vi "T2Mode_Acquisition_inertiaMotor.vi"() -> ()   [LabVIEW 2023]
uses:
  Types/MH_InputChannel.ctl
  Types/MH_UIThread_Cmds_T2.ctl
  cascorr/Multiharp/Types/MH_UIThread_Data_T2.ctl
  _lib/PQ/MultiHarp/MH_InitInfo.ctl
  Types/MH_SetInpChanData.ctl
  Types/MH_SetInpChanCmds.ctl
  _lib/PQ/MultiHarp/MH_RefSource.ctl
  _lib/PQ/MultiHarp/MH_MeasMode.ctl
  <vilib>/Utility/error.llb/DialogType.ctl
  <vilib>/Utility/error.llb/Error Cluster From Error Code.vi
  _lib/PQ/MultiHarp/MH_LibVersion_global.vi
  _lib/PQ/MultiHarp/mhlib_x86_x64_UIThread.llb/MH_DllPath_global.vi
  <vilib>/ErrorRing/Error Ring.xnode
panel:
  in  "Refresh(ms)":u32=500
  out "Waveform Chart":dbl[][](graph)
  in  "Monitor Range":i32=40
  in  "Path":path
  in  "FileName 2":string
  in  "Number of Acquisitions":i32=1 min=1 step=1
  out "x*y":dbl
  out "HistoGraph":T1(graph)={0.0, "Resolution"=0.08, "Histograms"=[]}
  in  "Run continuously":enum32{"Running Mode", "Item 1"}(radio) caption="Acquisition"
  in  "Start":bool
  in  "Scale":enum32{"Item 0", "Item 1"}(radio)
  out "CountRates":i32[](graph)
  in  "AllChannels":T2={"Enable"=TRUE, "Offset"=0, "Level"=20, "Edge"=0, "DeadTime"=1000, "UseDeadTime"=FALSE, "SetEnableAllChan"=TRUE, "SetEdgeAllChan"=TRUE, "SetLevelAllChan"=TRUE, "SetOffsetAllChan"=TRUE, "SetUseDTAllChan"=TRUE, "SetDeadTAllChan"=TRUE} {"DeadTime" min=800 max=160000 step=1; "Edge" items=["falling", "rising"]; "Offset" min=-100000 max=100000 step=10; "Level" min=-1200 max=1200 step=1}
  in  "HistoLength":i32(ring)=6 caption="Num Bins" items=["1024", "2048", "4096", "8192", "16384", "32768", "65536"]
  in  "OvlLevel":u32=4294967295 caption="Ovl.Level" min=1 step=1
  in  "StopOvl.":bool=TRUE
  in  "AcqTime":i32=1000 caption="Acqu.           ms" min=1 max=3600000 step=1
  in  "Binning":i32(ring) caption="Resol.            ps" items=["10", "20", "40", "80", "160", "320", "640", "1280", "2560", "5120", "10240", "20480", "40960", "81920", "163840", "327680", "655360", "1310720", "2621440", "5242880", "10485760", "20971520", "41943040"]
  in  "HistoOffset":i32 caption="Offset            ns" min=0 max=100000000 step=1
  in  "Acquire":bool
  in  "stop":bool
  in  "SyncDeadTime":i32=1000 caption="Dead T.   ps" min=800 max=160000 step=1
  in  "UseDeadTime":bool caption="Use DT."
  in  "SyncEdge":i32(ring) caption="Edge" items=["falling", "rising"]
  in  "SyncDivider":i32(ring) caption="Divider" items=["1", "2", "4", "8", "16"]
  in  "SyncOffset":i32 caption="Offset      ps" min=-100000 max=100000 step=10
  in  "SyncLevel":i32=-100 caption="Level      mV" min=-1200 max=1200 step=1
  in  "Channels":T3[](array[typedef])=[{"Name"="Inp.Chan 1", "Enable"=TRUE, "Edge"=0, "Level"=-100, "Offset"=0, "UseDeadTime"=FALSE, "DeadTime"=1000}, {"Name"="Inp.Chan 2", "Enable"=TRUE, "Edge"=0, "Level"=-100, "Offset"=0, "UseDeadTime"=FALSE, "DeadTime"=1000}, {"Name"="Inp.Chan 3", "Enable"=TRUE, "Edge"=0, "Level"=-100, "Offset"=0, "UseDeadTime"=FALSE, "DeadTime"=1000}, {"Name"="Inp.Chan 4", "Enable"=TRUE, "Edge"=0, "Level"=-100, "Offset"=0, "UseDeadTime"=FALSE, "DeadTime"=1000}, {"Name"="Inp.Chan 5", "Enable"=TRUE, "Edge"=0, "Level"=-100, "Offset"=0, "UseDeadTime"=FALSE, "DeadTime"=1000}, {"Name"="Inp.Chan 6", "Enable"=TRUE, "Edge"=0, "Level"=-100, "Offset"=0, "UseDeadTime"=FALSE, "DeadTime"=1000}, {"Name"="Inp.Chan 7", "Enable"=TRUE, "Edge"=0, "Level"=-100, "Offset"=0, "UseDeadTime"=FALSE, "DeadTime"=1000}, {"Name"="Inp.Chan 8", "Enable"=TRUE, "Edge"=0, "Level"=-100, "Offset"=0, "UseDeadTime"=FALSE, "DeadTime"=1000}, {"Name"="Inp.Chan 9", "Enable"=TRUE, "Edge"=0, "Level"=-100, "Offset"=0, "UseDeadTime"=FALSE, "DeadTime"=1000}, {"Name"="Inp.Chan 10", "Enable"=TRUE, "Edge"=0, "Level"=-100, "Offset"=0, "UseDeadTime"=FALSE, "DeadTime"=1000}, {"Name"="Inp.Chan 11", "Enable"=TRUE, "Edge"=0, "Level"=-100, "Offset"=0, "UseDeadTime"=FALSE, "DeadTime"=1000}, {"Name"="Inp.Chan 12", "Enable"=TRUE, "Edge"=0, "Level"=-100, "Offset"=0, "UseDeadTime"=FALSE, "DeadTime"=1000}, {"Name"="Inp.Chan 13", "Enable"=TRUE, "Edge"=0, "Level"=-100, "Offset"=0, "UseDeadTime"=FALSE, "DeadTime"=1000}, {"Name"="Inp.Chan 14", "Enable"=TRUE, "Edge"=0, "Level"=-100, "Offset"=0, "UseDeadTime"=FALSE, "DeadTime"=1000}, {"Name"="Inp.Chan 15", "Enable"=TRUE, "Edge"=0, "Level"=-100, "Offset"=0, "UseDeadTime"=FALSE, "DeadTime"=1000}, {"Name"="Inp.Chan 16", "Enable"=TRUE, "Edge"=0, "Level"=-100, "Offset"=0, "UseDeadTime"=FALSE, "DeadTime"=1000}] {"DeadTime" min=800 max=160000 step=1; "Edge" items=["falling", "rising"]; "Offset" min=-100000 max=100000 step=10; "Level" min=-1200 max=1200 step=1}
  out "SyncRate":string="Sync Rate: 4999950 cps\n"
  out "OverFlow":bool caption="Overflow:"
  out "Status":string="Readout Rate: 8.6 Hz\t\tTotal Counts:\t\tCh. 1: 0 cnts.\t\tCh. 2: 1962112 cnts.\t\tCh. 3: 0 cnts.\t\tCh. 4: 1962112 cnts.\t\tCh. 5: 0 cnts.\t\tCh. 6: 1962112 cnts.\t\tCh. 7: 0 cnts.\t\tCh. 8: 1962112 cnts.\t\tCh. 9: 1962113 cnts.\t\tCh.10: 0 cnts.\t\tCh.11: 1962113 cnts.\t\tCh.12: 0 cnts.\t\tCh.13: 1962113 cnts.\t\tCh.14: 0 cnts.\t\tCh.15: 1962113 cnts.\t\tCh.16: 1962113 cnts.\t\t"
  # "Single Counts"
  # "Coincidences vs time"
  # "Coincidences vs delay"
  # "Acquisition Options"
  # "Acquire Data"
  # "Piezo"
  # "Stage piezo"
  # "Scan"
  # "Jog"
  # "All Channels"
  # "Sync"
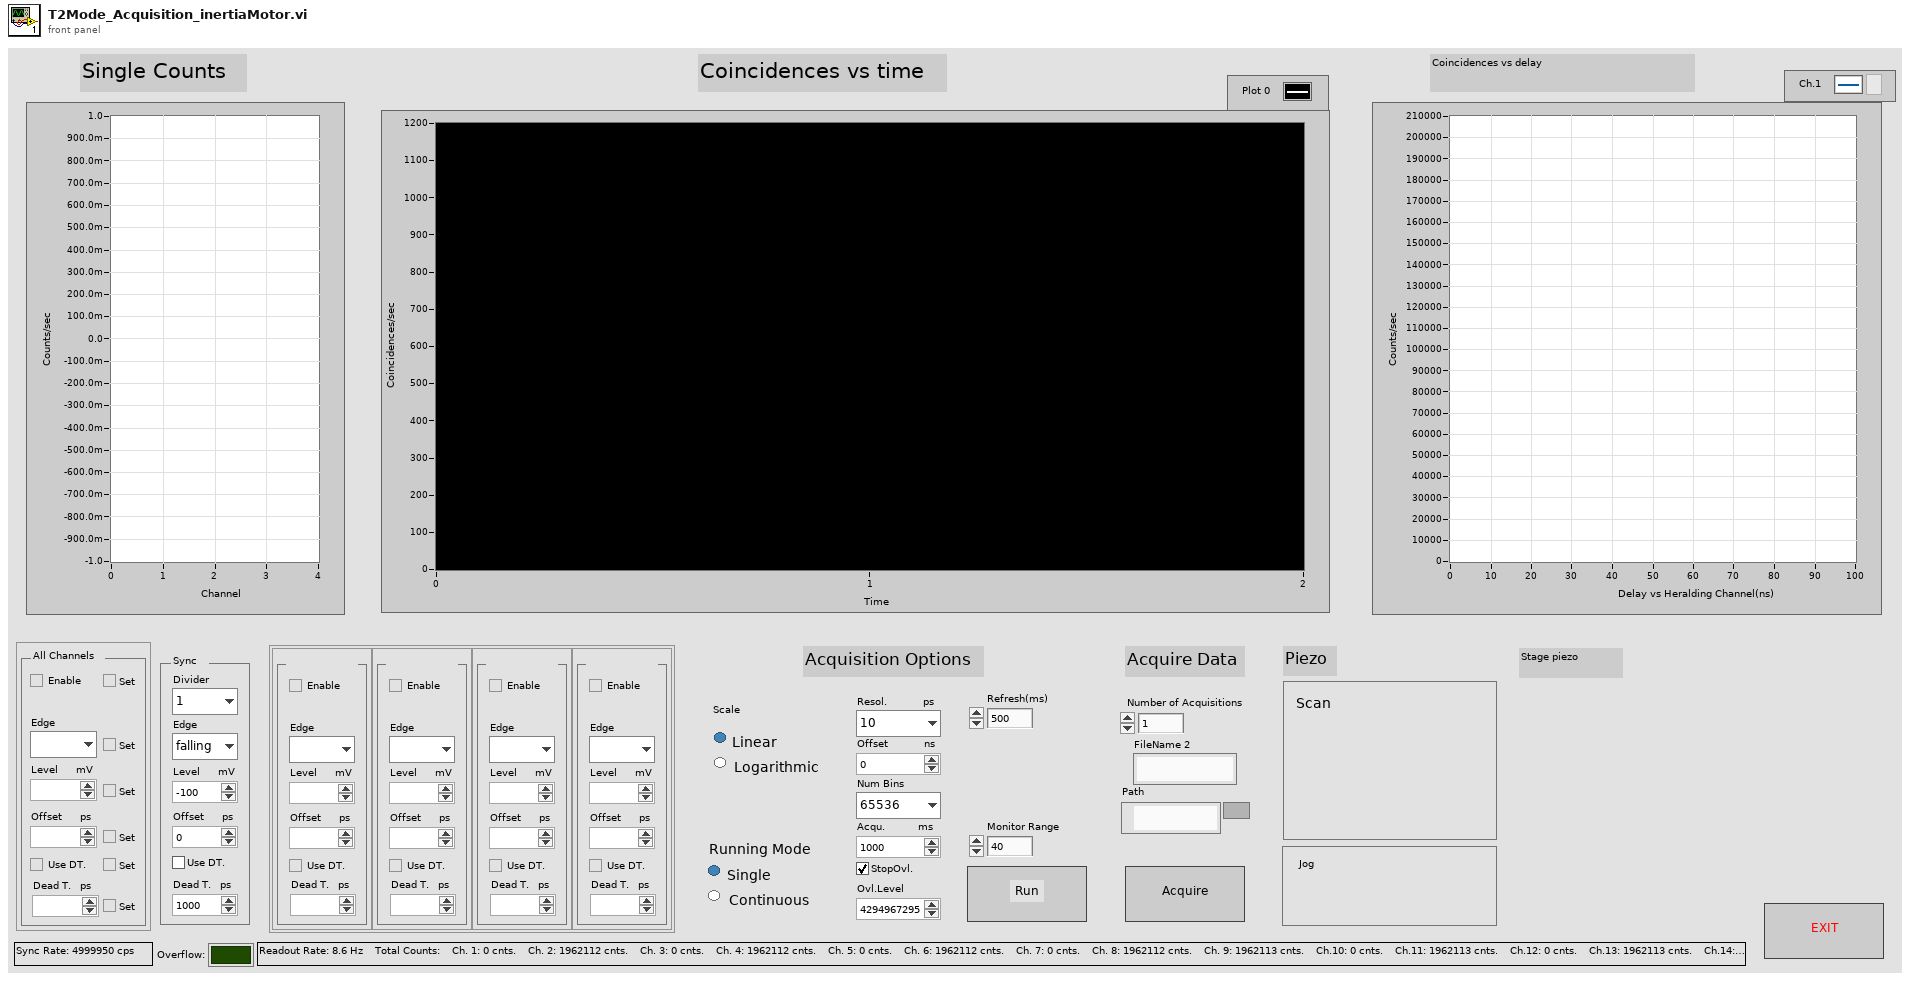
[diagram p1: front panel]
types:
  T1 = cluster{dbl, "Resolution":dbl, "Histograms":u32[][]}
  T2 = cluster{"Enable":bool, "Offset":i32, "Level":i32, "Edge":i32, "DeadTime":i32, "UseDeadTime":bool, "SetEnableAllChan":bool, "SetEdgeAllChan":bool, "SetLevelAllChan":bool, "SetOffsetAllChan":bool, "SetUseDTAllChan":bool, "SetDeadTAllChan":bool}
  T3 = typedef "MH_InputChannel.ctl" = cluster{"Name":string, "Enable":bool, "Edge":i32, "Level":i32, "Offset":i32, "UseDeadTime":bool, "DeadTime":i32}
  T4 = typedef "MH_UIThread_Data_T2.ctl" = cluster{"Init Info":T5, "DevIdx":i32, "SyncDivider":i32, "SyncOffset":i32, "SyncLevel":i32, "Channels":T3[], "CurrentChannels":i32[], "AcqTime":i32, "Binning":i32, "HistoOffset":i32, "HistoLen":i32, "StopOvl.":bool, "OvlLevel":u32, "SyncEdge":i32, "StartMeas":bool, "HistoLength":i32, "Resolution":dbl, "Run cont.":bool, "Status":string, "SyncRate":i32, "BitShift":i32, "HistoAcqTime":dbl, "SyncRateStart":i32, "UseDeadTime":bool, "SyncDeadTime":i32, "SetInpChan":T6[], "max value":u32[], "CoincidenceArray":dbl[][], "AcqTime 2":i32, "Fourier Transform":cluster{dbl, dbl, dbl[]}[], "fCh1":dbl[], "fCh2":dbl[], "fCh3":dbl[], "Refresh Rate":dbl, "HistoGraphOut":cluster{dbl, "Resolution":dbl, "Histograms":u32[][]}, "CountRates":i32[]}
  T5 = typedef "MH_InitInfo.ctl" = cluster{"Library Version":string, "Serial No.":string, "Model":string, "Partnum":string, "Version":string, "features":i32, "nchannels":i32, "Base Resolution":dbl, "Bin Steps":i32}
  T6 = typedef "MH_SetInpChanData.ctl" = cluster{"Channel":i32, "Cmds":T7[], "Changed":cluster{"Name":bool, "Enable":bool, "Edge":bool, "Level":bool, "Offset":bool, "UseDeadTime":bool, "DeadTime":bool}}
  T7 = typedef "MH_SetInpChanCmds.ctl" = enum16{"SetInpChanEnable", "SetInpChanOffset", "SetInpChanDeadTime", "SetInpChanTrg"}
  T8 = typedef "MH_UIThread_Cmds_T2.ctl" = enum16{"Idle", "Init", "SetInpChan", "SetSyncDivider", "SetSyncTrg", "SetSyncOffset", "SetSyncDeadTime", "SetBinning", "SetHistoOffset", "SetHistoLen", "SetStopOvl", "SetBitShift", "SetHistoAcqTime", "GetRates", "GetAllRates", "StartMeas", "StopMeas", "AbortMeas", "GetResolution", "GetHistos", "GetAllHistos", "ReadFiFo", "WriteStatus", "Resize", "EnableControls", "DisableControls", "Error", "Exit", "Acquire", "InitAcquisition"}
  T9 = enum8{"Enabled", "Disabled", "Disabled and Grayed Out"}
  T10 = typedef "MH_InputChannel2.ctl" = cluster{"Name":string, "Enable":bool, "Edge":i32, "Level":i32, "Offset":i32, "UseDeadTime":bool, "DeadTime":i32}
  T11 = cluster{"[0]":bool, "[1]":bool, "[2]":bool, "[3]":bool, "[4]":bool, "[5]":bool}
  T12 = typedef "MH_MeasMode.ctl" = i32
  T13 = typedef "MH_RefSource.ctl" = enum16{"INTERNAL", "EXTERNAL_10MHZ", "WR_MASTER_GENERIC", "WR_SLAVE_GENERIC", "WR_GRANDM_GENERIC", "EXTN_GPS_PPS", "EXTN_GPS_PPS_UART", "WR_MASTER_MHARP", "WR_SLAVE_MHARP", "WR_GRANDM_MHARP"}
  T14 = cluster{dbl, "Resolution":dbl, "Histogram":u32[][]}
  T15 = typedef "DialogType.ctl" = u16
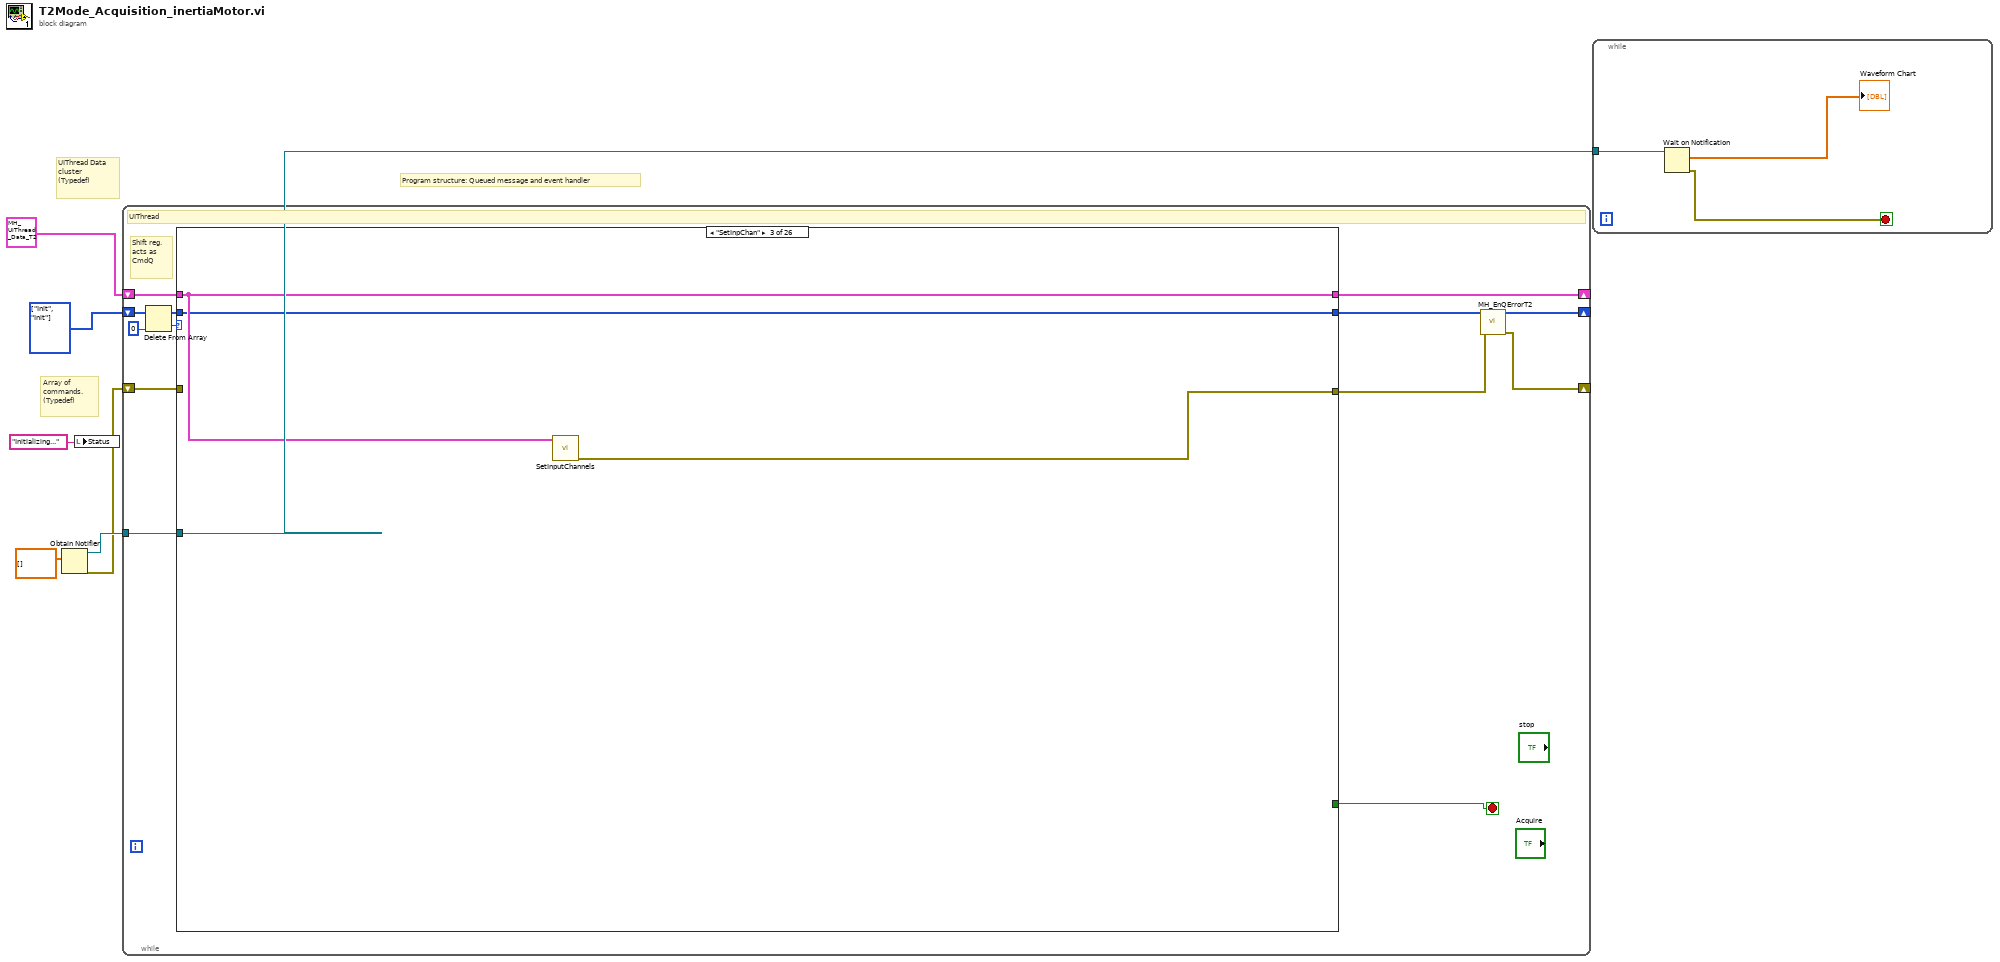
[diagram p0: block diagram]
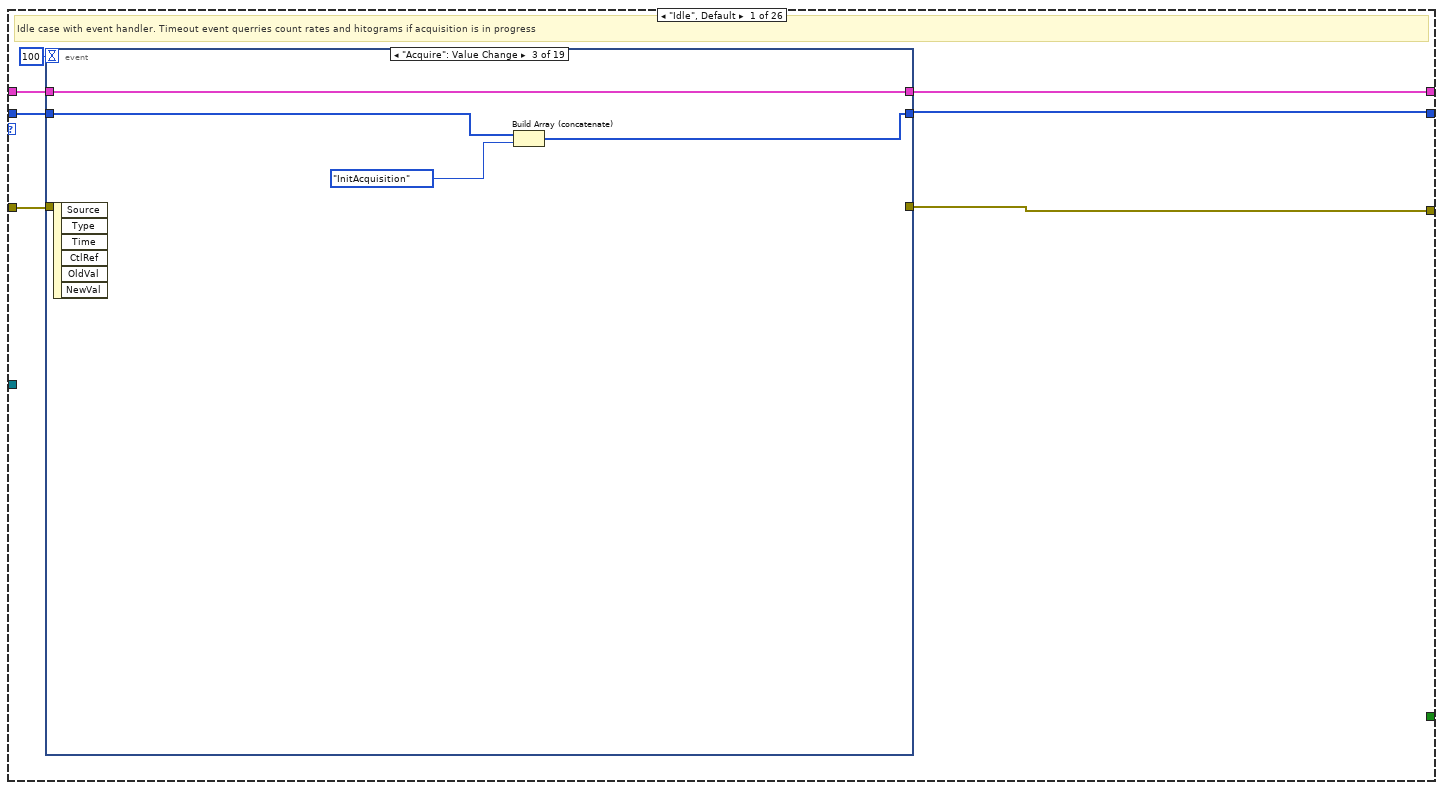
[diagram p2: hidden frame]
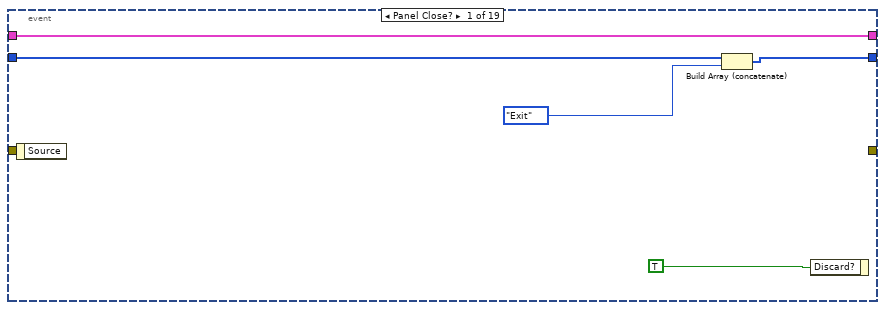
[diagram p3: hidden frame]
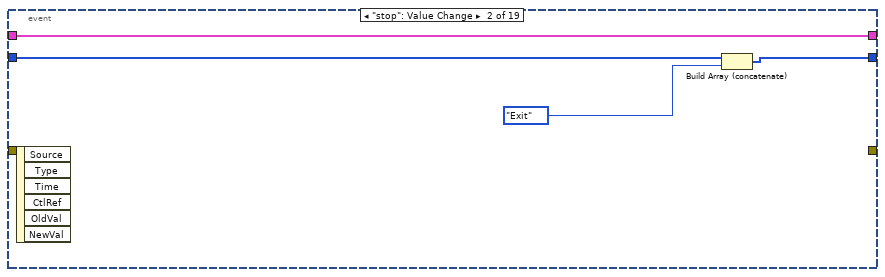
[diagram p4: hidden frame]
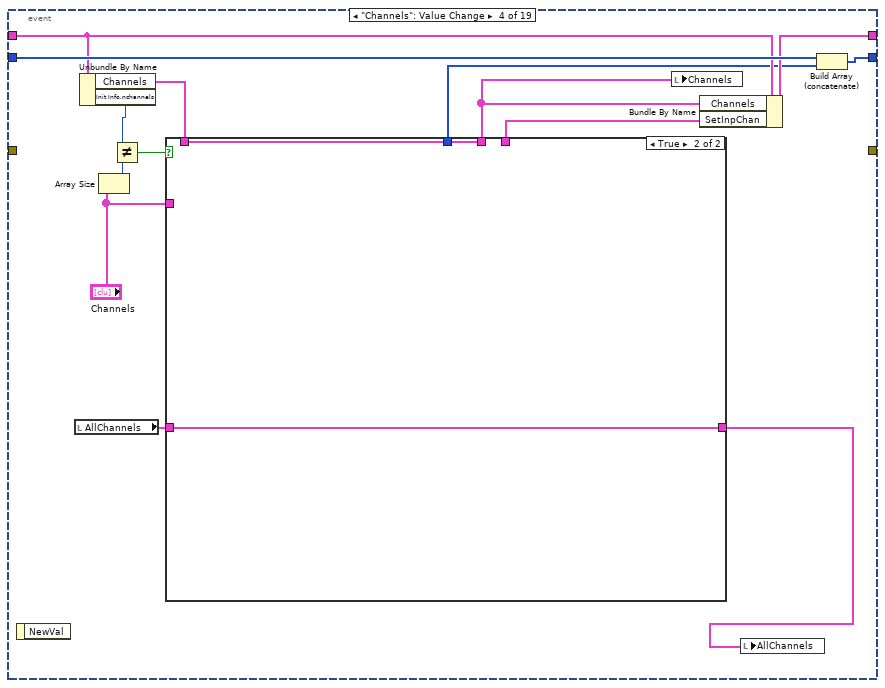
[diagram p5: hidden frame]
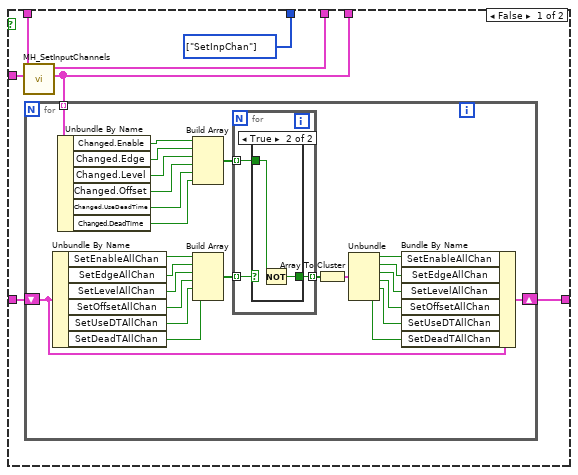
[diagram p6: hidden frame]
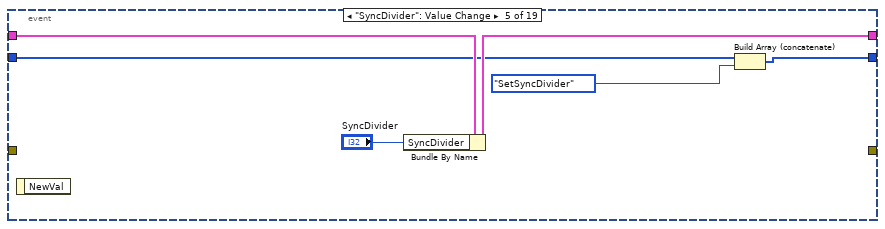
[diagram p8: hidden frame]
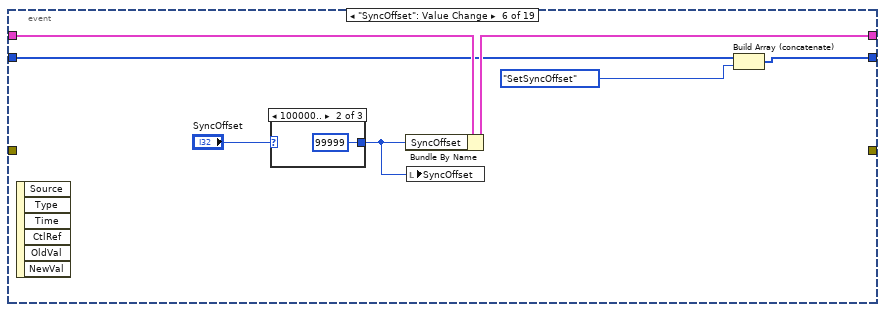
[diagram p9: hidden frame]
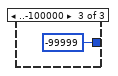
[diagram p11: hidden frame]
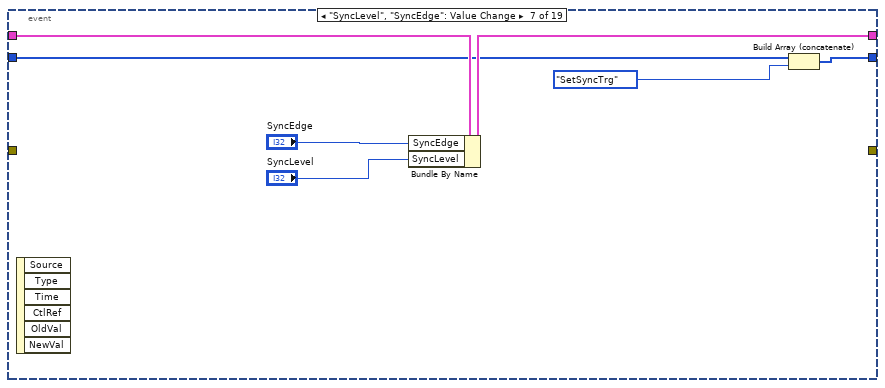
[diagram p12: hidden frame]
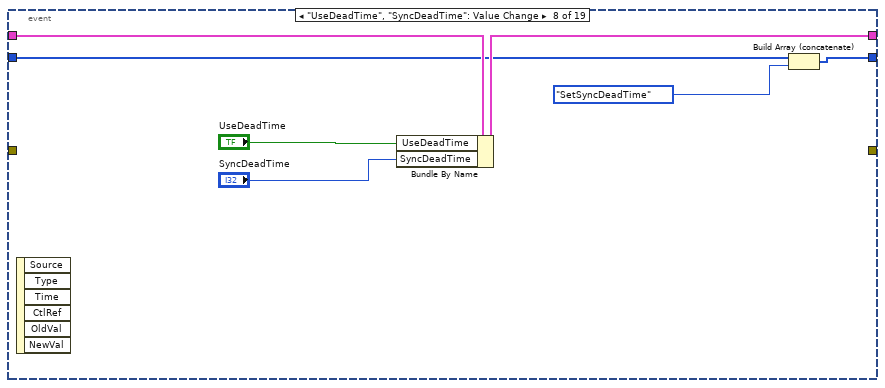
[diagram p13: hidden frame]
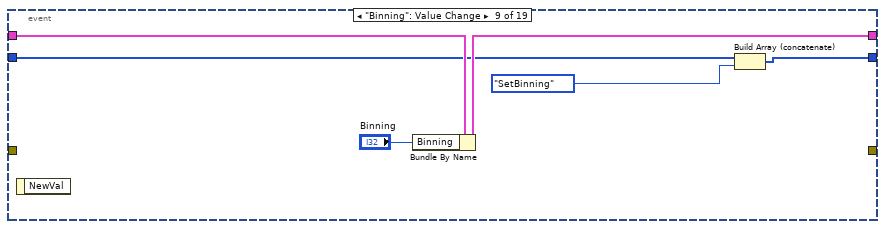
[diagram p14: hidden frame]
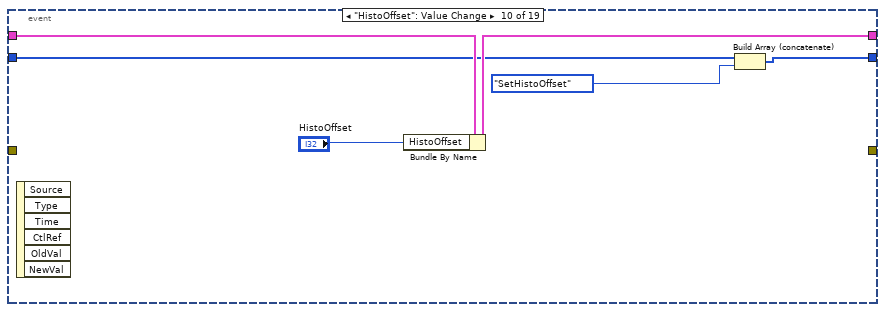
[diagram p15: hidden frame]
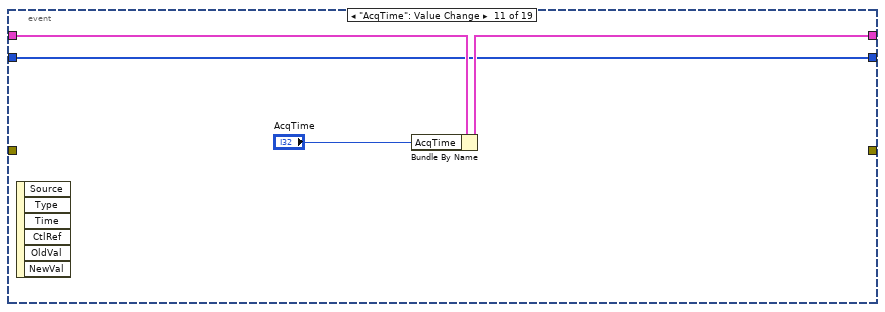
[diagram p16: hidden frame]
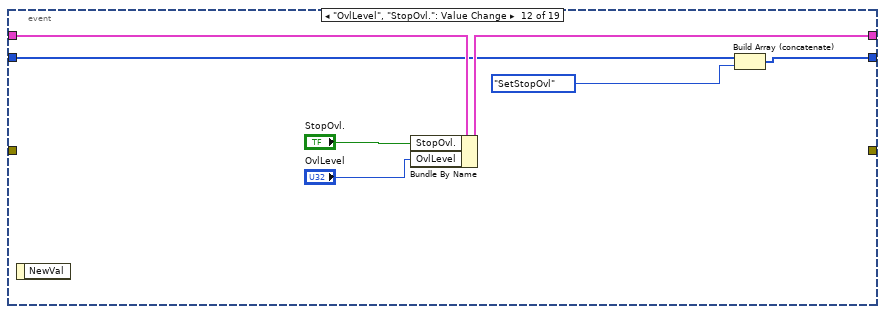
[diagram p17: hidden frame]
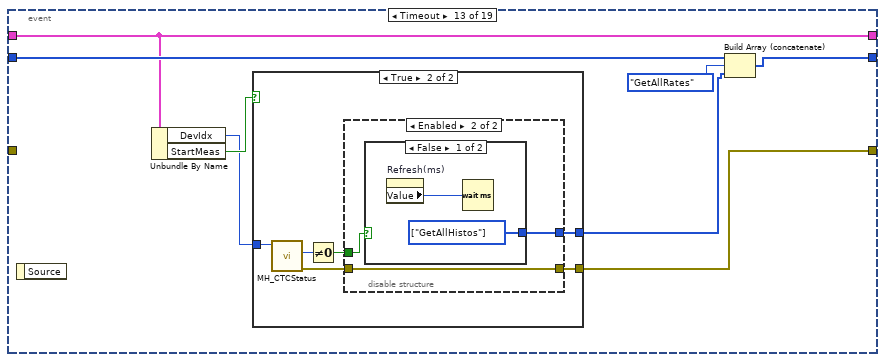
[diagram p18: hidden frame]
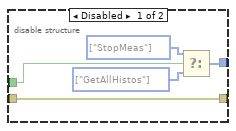
[diagram p20: hidden frame]
diagram:
  w6 = T8[] [enum."Init", enum."Init"] items=["Idle", "Init", "SetInpChan", "SetSyncDivider", "SetSyncTrg", "SetSyncOffset", "SetSyncDeadTime", "SetBinning", "SetHistoOffset", "SetHistoLen", "SetStopOvl", "SetBitShift", "SetHistoAcqTime", "GetRates", "GetAllRates", "StartMeas", "StopMeas", "AbortMeas", "GetResolution", "GetHistos", "GetAllHistos", "ReadFiFo", "WriteStatus", "Resize", "EnableControls", "DisableControls", "Error", "Exit", "Acquire", "InitAcquisition"]
  # "Array of commands.\n(Typedef)"
  # "Program structure: Queued message and event handler"
  # "UIThread Data cluster\n(Typedef)"
  n1 = Obtain Notifier(notification data type=dbl[][] [] ("element data type")) -> (notifier out=w2:refnum<notifier>, error out=w1:errorcluster)  [unwired: 3 in, 1 out]
  n2 = local write "Status"("Initializing..." ("Status")) -> ()
  n3 = while {
    shift-right: [w9] -> _
    shift-left: w6 -> [w15]
    shift-right: [w18] -> _
    shift-left: T4 {"Init Info"={"Library Version"="", "Serial No."="", "Model"="", "Partnum"="", "Version"="", "features"=0, "nchannels"=0, "Base Resolution"=0.0, "Bin Steps"=0}, "DevIdx"=0, "SyncDivider"=1, "SyncOffset"=0, "SyncLevel"=50, "Channels"=[], "CurrentChannels"=[], "AcqTime"=1, "Binning"=1, "HistoOffset"=1, "HistoLen"=1024, "StopOvl."=FALSE, "OvlLevel"=1024, "SyncEdge"=10, "StartMeas"=FALSE, "HistoLength"=0, "Resolution"=0.0, "Run cont."=FALSE, "Status"="", "SyncRate"=0, "BitShift"=0, "HistoAcqTime"=0.0, "SyncRateStart"=0, "UseDeadTime"=FALSE, "SyncDeadTime"=800, "SetInpChan"=[], "max value"=[], "CoincidenceArray"=[], "AcqTime 2"=1000, "Fourier Transform"=[], "fCh1"=[], "fCh2"=[], "fCh3"=[], "Refresh Rate"=0.0, "HistoGraphOut"={0.0, "Resolution"=0.08, "Histograms"=[]}, "CountRates"=[]} -> [w17]
    shift-right: [w10] -> _
    shift-left: w1 -> [w16]
    tunnel: w2 -> [w8]
    stop <- w19 stop-if-true
    # "Shift reg.\nacts as\nCmdQ"
    # "UIThread"
    n4 = Delete From Array(array=w15, index=0) -> (deleted portion=w13:T8, array with subset deleted=w12:T8[])  [unwired: 1 in]
    n5 = case shown="\"SetInpChan\"" w13 {
      tunnel: [_ _ _ _ _ _ _ _ _ _ _ _ _ _ _ _ _ _ _ _ _ _ _ TRUE _ _] -> w19
      tunnel: [w26 w289 w327 w330 w336 w348 w357 w364 w369 w372 w382 w393 w404 w420 w432 w446 w454 w474 w539 w563 w570 w582 w589 w599 w602 w612] -> w18
      tunnel: w17 -> [w25 w294 w327 w330 w336 w348 w357 w364 w369 w373 w382 w393 w404 w421 w433 w447 w455 w475 w539 w563 w570 w582 w589 w599 w602 w612]
      tunnel: [w22 w310 w326 w329 w335 w347 w356 w363 w368 w376 w381 w389 w403 w427 w435 w449 w456 w472 w535 _ _ _ _ w594 w603 w613] -> w11
      tunnel: w16 -> [w20 _ _ _ _ _ _ _ _ _ _ _ _ _ _ _ _ _ _ _ _ _ w590 w597 _ _]
      tunnel: w12 -> [w24 w309 w325 w328 w331 w337 w353 w360 w365 w370 w377 w383 w394 w423 w430 w444 w450 w458 w515 w561 w564 w576 _ w592 w609 w615]
      tunnel: w8 -> [_ _ _ _ _ _ _ _ _ _ _ _ _ _ _ _ _ w469 _ _ _ _ _ w593 _ _]
      tunnel: [w21 w260 w325 w328 w331 w337 w353 w358 w365 w370 w377 w383 w394 w418 w428 w442 w450 w458 w515 w561 w564 w576 w588 w592 w601 w611] -> w7
      frame "Idle", Default {
        # "Idle case with event handler. Timeout event querries count rates and hitograms if acquisition is in progress"
        n6 = event shown="[2] \"Acquire\": Value Change" {
          selector: _ -> [_ _ _ _ _ _ _ _ _ _ _ _ _ _ _ _ _ _ _]
          dyn-events: _ -> [_ _ _ _ _ _ _ _ _ _ _ _ _ _ _ _ _ _ _]
          timeout: 100 -> [_ _ _ _ _ _ _ _ _ _ _ _ _ _ _ _ _ _ _]
          tunnel: [w27 w32 w36 w40 w94 w100 w110 w117 w124 w130 w136 w140 w151 w172 w178 w186 w193 w196 w200] -> w21
          tunnel: [w30 w35 w39 w46 w98 w105 w115 w122 w128 w134 w138 w145 w153 w176 w180 w191 w195 w199 w204] -> w26
          tunnel: w25 -> [w30 w35 w39 w48 w99 w106 w116 w123 w129 w135 w139 w146 w153 w177 w181 w192 w195 w199 w205]
          tunnel: w24 -> [w29 w34 w38 w53 w96 w104 w113 w121 w127 w133 w136 w144 w154 w175 w183 w186 w193 w197 w210]
          tunnel: [_ _ _ _ _ _ _ _ _ _ _ _ w152 _ _ _ _ _ _] -> w22
          tunnel: w20 -> [_ _ _ _ _ _ _ _ _ _ _ _ _ _ _ _ _ _ _]
          event Panel Close? {
            n7 = event-data() -> ()  [unwired: 1 in, 1 out]
            n8 = Build Array (concatenate)(w29, MH_UIThread_Cmds_T2."Exit") -> (w27:T8[])
            n9 = event-data("Discard?"=TRUE) -> ()  [unwired: 1 in, 1 out]
          }
          event "stop": Value Change {
            n10 = event-data() -> ()  [unwired: 1 in, 6 out]
            n11 = Build Array (concatenate)(w34, MH_UIThread_Cmds_T2."Exit") -> (w32:T8[])
          }
          event "Acquire": Value Change {
            n12 = event-data() -> ()  [unwired: 1 in, 6 out]
            n13 = Build Array (concatenate)(w38, MH_UIThread_Cmds_T2."InitAcquisition") -> (w36:T8[])
          }
          event "Channels": Value Change {
            n14 = event-data() -> ()  [unwired: 1 in, 1 out]
            n15 = local read "AllChannels"() -> (w42:T2)
            n16 = Unbundle By Name(w48) -> ("Channels"=w49:T3[], "Init Info.nchannels"=w52:i32)
            n17 = Array Size(array="Channels") -> (size(s)=w51:i32)
            n18 = Not Equal?(x=w52, y=w51) -> (x != y?=w50:bool)
            n19 = case shown="True" w50 {
              tunnel: "Channels" -> [w59 _]
              tunnel: [w58 w93] -> w47
              tunnel: w49 -> [w60 w93]
              tunnel: [w56 _] -> w45
              tunnel: [w57 _] -> w43
              tunnel: w42 -> [w55 w92]
              tunnel: [w54 w92] -> w41
              frame False {
                w57 = T8[] [enum."SetInpChan"] items=["Idle", "Init", "SetInpChan", "SetSyncDivider", "SetSyncTrg", "SetSyncOffset", "SetSyncDeadTime", "SetBinning", "SetHistoOffset", "SetHistoLen", "SetStopOvl", "SetBitShift", "SetHistoAcqTime", "GetRates", "GetAllRates", "StartMeas", "StopMeas", "AbortMeas", "GetResolution", "GetHistos", "GetAllHistos", "ReadFiFo", "WriteStatus", "Resize", "EnableControls", "DisableControls", "Error", "Exit", "Acquire", "InitAcquisition"] ("array")
                n20 = call "MH_SetInputChannels.vi"("Channels new"=w59, "Channels old"=w60) -> ("SetInpChan"=w56:T6[], "Channels"=w58:T10[])  [unwired: 8 in]
                n21 = for {
                  tunnel: w56 -> [w85] mode=indexing
                  shift-right: [w67] -> w54
                  shift-left: w55 -> [w69]
                  n22 = Unbundle By Name(w69) -> ("SetEnableAllChan"=w78:bool, "SetEdgeAllChan"=w77:bool, "SetLevelAllChan"=w76:bool, "SetOffsetAllChan"=w75:bool, "SetUseDTAllChan"=w74:bool, "SetDeadTAllChan"=w73:bool)
                  n23 = Unbundle By Name(w85) -> ("Changed.Enable"=w84:bool, "Changed.Edge"=w83:bool, "Changed.Level"=w82:bool, "Changed.Offset"=w81:bool, "Changed.UseDeadTime"=w80:bool, "Changed.DeadTime"=w79:bool)
                  n24 = Build Array(w84, w83, w82, w81, w80, w79) -> (w71:bool[])
                  n25 = Build Array(w78, w77, w76, w75, w74, w73) -> (w72:bool[])
                  n26 = for {
                    tunnel: w72 -> [w88] mode=indexing
                    tunnel: w71 -> [w86] mode=indexing
                    tunnel: [w87] -> w70 mode=indexing
                    n27 = case shown="True" w88 {
                      selector: w88 -> [w89 _]
                      tunnel: [w89 w90] -> w87
                      tunnel: w86 -> [_ w91]
                      frame False {
                      }
                      frame True {
                        n28 = Not(x=w91) -> (.not. x?=w90:bool)
                      }
                    }
                  }
                  n29 = Array To Cluster(array=w70) -> (cluster=w68:T11)
                  n30 = Unbundle(w68) -> ("[0]"=w66:bool, "[1]"=w65:bool, "[2]"=w64:bool, "[3]"=w63:bool, "[4]"=w62:bool, "[5]"=w61:bool)
                  n31 = Bundle By Name(cluster=w69, "SetEnableAllChan"=w66, "SetEdgeAllChan"=w65, "SetLevelAllChan"=w64, "SetOffsetAllChan"=w63, "SetUseDTAllChan"=w62, "SetDeadTAllChan"=w61) -> (w67:T2)
                }
              }
              frame True {
              }
            }
            n32 = local write "Channels"(w47) -> ()
            n33 = Bundle By Name(cluster=w48, "Channels"=w47, "SetInpChan"=w45) -> (w46:T4)
            n34 = local write "AllChannels"(w41) -> ()
            n35 = Build Array (concatenate)(w53, w43) -> (w40:T8[])
          }
          event "SyncDivider": Value Change {
            n36 = event-data() -> ()  [unwired: 1 in, 1 out]
            n37 = Bundle By Name(cluster=w99, "SyncDivider"="SyncDivider") -> (w98:T4)
            n38 = Build Array (concatenate)(w96, MH_UIThread_Cmds_T2."SetSyncDivider") -> (w94:T8[])
          }
          event "SyncOffset": Value Change {
            n39 = event-data() -> ()  [unwired: 1 in, 6 out]
            n40 = case shown="100000.." "SyncOffset" {
              selector: "SyncOffset" -> [w107 _ _]
              tunnel: [w107 99999 ("SyncOffset") -99999 ("SyncOffset")] -> w101
              frame Default {
              }
              frame 100000.. {
              }
              frame ..-100000 {
              }
            }
            n41 = Bundle By Name(cluster=w106, "SyncOffset"=w101) -> (w105:T4)
            n42 = local write "SyncOffset"(w101) -> ()
            n43 = Build Array (concatenate)(w104, MH_UIThread_Cmds_T2."SetSyncOffset") -> (w100:T8[])
          }
          event "SyncLevel", "SyncEdge": Value Change {
            n44 = event-data() -> ()  [unwired: 1 in, 6 out]
            n45 = Bundle By Name(cluster=w116, "SyncEdge"="SyncEdge", "SyncLevel"="SyncLevel") -> (w115:T4)
            n46 = Build Array (concatenate)(w113, MH_UIThread_Cmds_T2."SetSyncTrg") -> (w110:T8[])
          }
          event "UseDeadTime", "SyncDeadTime": Value Change {
            n47 = event-data() -> ()  [unwired: 1 in, 6 out]
            n48 = Bundle By Name(cluster=w123, "UseDeadTime"="UseDeadTime", "SyncDeadTime"="SyncDeadTime") -> (w122:T4)
            n49 = Build Array (concatenate)(w121, MH_UIThread_Cmds_T2."SetSyncDeadTime") -> (w117:T8[])
          }
          event "Binning": Value Change {
            n50 = event-data() -> ()  [unwired: 1 in, 1 out]
            n51 = Bundle By Name(cluster=w129, "Binning"="Binning") -> (w128:T4)
            n52 = Build Array (concatenate)(w127, MH_UIThread_Cmds_T2."SetBinning") -> (w124:T8[])
          }
          event "HistoOffset": Value Change {
            n53 = event-data() -> ()  [unwired: 1 in, 6 out]
            n54 = Bundle By Name(cluster=w135, "HistoOffset"="HistoOffset") -> (w134:T4)
            n55 = Build Array (concatenate)(w133, MH_UIThread_Cmds_T2."SetHistoOffset") -> (w130:T8[])
          }
          event "AcqTime": Value Change {
            n56 = event-data() -> ()  [unwired: 1 in, 6 out]
            n57 = Bundle By Name(cluster=w139, "AcqTime"="AcqTime") -> (w138:T4)
          }
          event "OvlLevel", "StopOvl.": Value Change {
            n58 = event-data() -> ()  [unwired: 1 in, 1 out]
            n59 = Bundle By Name(cluster=w146, "StopOvl."="StopOvl.", "OvlLevel"="OvlLevel") -> (w145:T4)
            n60 = Build Array (concatenate)(w144, MH_UIThread_Cmds_T2."SetStopOvl") -> (w140:T8[])
          }
          event Timeout {
            n61 = event-data() -> ()  [unwired: 1 in, 1 out]
            n62 = Unbundle By Name(w153) -> ("DevIdx"=w148:i32, "StartMeas"=w149:bool)
            n63 = case shown="True" w149 {
              tunnel: w148 -> [_ w160]
              tunnel: [_ w158] -> w147
              tunnel: [_ w155] -> w152
              frame False {
              }
              frame True {
                n64 = call "MH_CTCStatus.vi"("devidx"=w160) -> ("error out"=w156:errorcluster, "ctcstatus"=w159:i32)  [unwired: 8 in, 1 out]
                n65 = Not Equal To 0?(x=w159) -> (x != 0?=w157:bool)
                n66 = disable-structure shown="Enabled" {
                  disable-tunnel: [w165 w167] -> w158
                  disable-tunnel: w157 -> [w163 w168]
                  disable-tunnel: w156 -> [w161 w166]
                  disable-tunnel: [w161 w166] -> w155
                  frame Disabled {
                    w162 = T8[] [enum."GetAllHistos"] items=["Idle", "Init", "SetInpChan", "SetSyncDivider", "SetSyncTrg", "SetSyncOffset", "SetSyncDeadTime", "SetBinning", "SetHistoOffset", "SetHistoLen", "SetStopOvl", "SetBitShift", "SetHistoAcqTime", "GetRates", "GetAllRates", "StartMeas", "StopMeas", "AbortMeas", "GetResolution", "GetHistos", "GetAllHistos", "ReadFiFo", "WriteStatus", "Resize", "EnableControls", "DisableControls", "Error", "Exit", "Acquire", "InitAcquisition"]
                    w164 = T8[] [enum."StopMeas"] items=["Idle", "Init", "SetInpChan", "SetSyncDivider", "SetSyncTrg", "SetSyncOffset", "SetSyncDeadTime", "SetBinning", "SetHistoOffset", "SetHistoLen", "SetStopOvl", "SetBitShift", "SetHistoAcqTime", "GetRates", "GetAllRates", "StartMeas", "StopMeas", "AbortMeas", "GetResolution", "GetHistos", "GetAllHistos", "ReadFiFo", "WriteStatus", "Resize", "EnableControls", "DisableControls", "Error", "Exit", "Acquire", "InitAcquisition"]
                    n67 = Select(t=w164, s=w163, f=w162) -> (s? t:f=w165:T8[])
                  }
                  frame Enabled {
                    n68 = case shown="False" w168 {
                      tunnel: [w170 w171] -> w167
                      frame False {
                        w170 = T8[] [enum."GetAllHistos"] items=["Idle", "Init", "SetInpChan", "SetSyncDivider", "SetSyncTrg", "SetSyncOffset", "SetSyncDeadTime", "SetBinning", "SetHistoOffset", "SetHistoLen", "SetStopOvl", "SetBitShift", "SetHistoAcqTime", "GetRates", "GetAllRates", "StartMeas", "StopMeas", "AbortMeas", "GetResolution", "GetHistos", "GetAllHistos", "ReadFiFo", "WriteStatus", "Resize", "EnableControls", "DisableControls", "Error", "Exit", "Acquire", "InitAcquisition"]
                        n69 = property on="Refresh(ms)" class="DigNum (strict)"() -> ("Value"=w169:u32)  [unwired: 2 in, 2 out]
                        n70 = Wait (ms)(milliseconds to wait=w169) -> ()  [unwired: 1 out]
                      }
                      frame True {
                        w171 = T8[] [enum."StopMeas"] items=["Idle", "Init", "SetInpChan", "SetSyncDivider", "SetSyncTrg", "SetSyncOffset", "SetSyncDeadTime", "SetBinning", "SetHistoOffset", "SetHistoLen", "SetStopOvl", "SetBitShift", "SetHistoAcqTime", "GetRates", "GetAllRates", "StartMeas", "StopMeas", "AbortMeas", "GetResolution", "GetHistos", "GetAllHistos", "ReadFiFo", "WriteStatus", "Resize", "EnableControls", "DisableControls", "Error", "Exit", "Acquire", "InitAcquisition"]
                      }
                    }
                  }
                }
              }
            }
            n71 = Build Array (concatenate)(w154, MH_UIThread_Cmds_T2."GetAllRates", w147) -> (w151:T8[])
          }
          event "HistoLength": Value Change {
            n72 = event-data() -> ()  [unwired: 1 in, 6 out]
            n73 = Bundle By Name(cluster=w177, "HistoLen"="HistoLength") -> (w176:T4)
            n74 = Build Array (concatenate)(w175, MH_UIThread_Cmds_T2."SetHistoLen") -> (w172:T8[])
          }
          event "Start": Value Change {
            n75 = event-data() -> ()  [unwired: 1 in, 1 out]
            n76 = Select(t=MH_UIThread_Cmds_T2."StartMeas", s="Start", f=MH_UIThread_Cmds_T2."AbortMeas") -> (s? t:f=w182:T8)
            n77 = Bundle By Name(cluster=w181, "StartMeas"="Start") -> (w180:T4)
            n78 = Build Array (concatenate)(w183, w182) -> (w178:T8[])
          }
          event "Run continuously": Value Change {
            n79 = event-data() -> ()  [unwired: 1 in, 1 out]
            n80 = Number To Boolean Array(number="Run continuously") -> (Boolean array=w189:bool[])
            n81 = Delete From Array(array=w189, index=0) -> (deleted portion=w187:bool)  [unwired: 1 in, 1 out]
            n82 = Bundle By Name(cluster=w192, "Run cont."=w187) -> (w191:T4)
          }
          event "Scale": Value Change {
            n83 = event-data() -> ()  [unwired: 1 in, 1 out]
            n84 = property on="HistoGraph" class="WFGraph (strict)"("YScale.Mapping Mode"="Scale") -> ()  [unwired: 2 in, 2 out]
          }
          event Panel Resize {
            n85 = event-data() -> ()  [unwired: 1 in, 1 out]
            n86 = Build Array (concatenate)(w197, MH_UIThread_Cmds_T2."Resize") -> (w196:T8[])
          }
          event "AllChannels": Value Change {
            w202 = T8[] [enum."SetInpChan"] items=["Idle", "Init", "SetInpChan", "SetSyncDivider", "SetSyncTrg", "SetSyncOffset", "SetSyncDeadTime", "SetBinning", "SetHistoOffset", "SetHistoLen", "SetStopOvl", "SetBitShift", "SetHistoAcqTime", "GetRates", "GetAllRates", "StartMeas", "StopMeas", "AbortMeas", "GetResolution", "GetHistos", "GetAllHistos", "ReadFiFo", "WriteStatus", "Resize", "EnableControls", "DisableControls", "Error", "Exit", "Acquire", "InitAcquisition"] ("array")
            n87 = event-data() -> ()  [unwired: 1 in, 1 out]
            n88 = local read "Channels"() -> (w209:T3[])
            n89 = for {
              tunnel: w209 -> [w213] mode=indexing
              tunnel: "AllChannels" -> [w212]
              tunnel: [w211] -> w207 mode=indexing
              n90 = Unbundle By Name(w212) -> ("SetEnableAllChan"=w214:bool, "SetEdgeAllChan"=w215:bool, "SetLevelAllChan"=w216:bool, "SetOffsetAllChan"=w217:bool, "SetUseDTAllChan"=w218:bool, "SetDeadTAllChan"=w219:bool)
              n91 = Build Array(w214, w215, w216, w217, w218, w219) -> (w220:bool[])
              n92 = for {
                tunnel: w220 -> [w225] mode=indexing
                shift-right: [w222] -> w211
                shift-left: w213 -> [w223]
                tunnel: w212 -> [w221]
                i -> [w224]
                n93 = case shown="True" w225 {
                  tunnel: w224 -> [_ w230]
                  tunnel: w221 -> [_ w229]
                  tunnel: w223 -> [w226 w228]
                  tunnel: [w226 w227] -> w222
                  frame False {
                  }
                  frame True {
                    n94 = case shown="Default" w230 {
                      tunnel: w229 -> [w234 w238 w242 w247 w254 w258 _]
                      tunnel: w228 -> [w233 w237 w241 w246 w253 w257 w259]
                      tunnel: [w231 w235 w239 w245 w251 w255 w259] -> w227
                      frame 0 {
                        n95 = Unbundle By Name(w234) -> ("Enable"=w232:bool)
                        n96 = Bundle By Name(cluster=w233, "Enable"=w232) -> (w231:T3)
                      }
                      frame 1 {
                        n97 = Unbundle By Name(w238) -> ("Edge"=w236:i32)
                        n98 = Bundle By Name(cluster=w237, "Edge"=w236) -> (w235:T3)
                      }
                      frame 2 {
                        n99 = Unbundle By Name(w242) -> ("Level"=w240:i32)
                        n100 = Bundle By Name(cluster=w241, "Level"=w240) -> (w239:T3)
                      }
                      frame 3 {
                        n101 = Unbundle By Name(w247) -> ("Offset"=w244:i32)
                        n102 = case shown="100000.." w244 {
                          selector: w244 -> [w248 _ _]
                          tunnel: [w248 99999 ("SyncOffset") -99999 ("SyncOffset")] -> w243
                          frame Default {
                          }
                          frame 100000.. {
                          }
                          frame ..-100000 {
                          }
                        }
                        n103 = Bundle By Name(cluster=w246, "Offset"=w243) -> (w245:T3)
                      }
                      frame 4 {
                        n104 = Unbundle By Name(w254) -> ("UseDeadTime"=w252:bool)
                        n105 = Bundle By Name(cluster=w253, "UseDeadTime"=w252) -> (w251:T3)
                      }
                      frame 5 {
                        n106 = Unbundle By Name(w258) -> ("DeadTime"=w256:i32)
                        n107 = Bundle By Name(cluster=w257, "DeadTime"=w256) -> (w255:T3)
                      }
                      frame Default {
                      }
                    }
                  }
                }
              }
            }
            n108 = Build Array (concatenate)(w210, w202) -> (w200:T8[])
            n109 = Unbundle By Name(w205) -> ("Channels"=w206:T3[])
            n110 = call "MH_SetInputChannels.vi"("Channels new"=w207, "Channels old"=w206) -> ("SetInpChan"=w203:T6[], "Channels"=w201:T10[])  [unwired: 8 in]
            n111 = local write "Channels"(w201) -> ()
            n112 = Bundle By Name(cluster=w205, "Channels"=w201, "SetInpChan"=w203) -> (w204:T4)
          }
        }
      }
      frame "Init" {
        w271 = 1000 ("SyncDeadTime")
        w272 = FALSE ("UseDeadTime")
        w274 = T12 0 items=["HIST"=0, "T2"=2, "T3"=3]  # Mode
        w283 = MH_RefSource."INTERNAL"  # refsource
        w297 = FALSE ("StartMeas")
        w298 = u32 4294967295 ("OvlLevel")
        w299 = TRUE ("StopOvl.")
        w300 = 0 ("HistoLen")
        w301 = 10000 ("AcqTime")
        w302 = 0 ("HistoOffset")
        w303 = 7 ("Binning")
        w304 = 20 ("SyncLevel")
        w305 = 1 ("SyncZeroX")
        w306 = -50000 ("SyncOffset")
        w307 = 0 ("SyncDivider")
        w308 = T8[] [enum."SetSyncDivider", enum."SetSyncOffset", enum."SetSyncTrg", enum."SetSyncDeadTime", enum."SetInpChan", enum."SetBinning", enum."SetHistoOffset", enum."SetHistoLen", enum."SetStopOvl", enum."Resize", enum."EnableControls", enum."WriteStatus"] items=["Idle", "Init", "SetInpChan", "SetSyncDivider", "SetSyncTrg", "SetSyncOffset", "SetSyncDeadTime", "SetBinning", "SetHistoOffset", "SetHistoLen", "SetStopOvl", "SetBitShift", "SetHistoAcqTime", "GetRates", "GetAllRates", "StartMeas", "StopMeas", "AbortMeas", "GetResolution", "GetHistos", "GetAllHistos", "ReadFiFo", "WriteStatus", "Resize", "EnableControls", "DisableControls", "Error", "Exit", "Acquire", "InitAcquisition"]
        # "Init HW"
        # "Set path to mhlib.dll"
        # "Init all FP controls and corresponding copy in UIThread Data cluster"
        # "EnQ list of commands"
        # "Array with Inp.Chan."
        # "Initialization: 1. Init HW -> get # of channels -> make array for Inp.Channels\n2. Init all FP controls and corresponding fields in UIThread Data cluster\n3. EnQ list of commands for further initialization"
        n113 = disable-structure shown="TARGET_TYPE==Windows, Default" {
          disable-tunnel: ["MHLib64" ("name or relative path") "MHLib" ("name or relative path")] -> w273
          frame condition #0 (active) {
          }
          frame condition #1 {
          }
        }
        n114 = xnode "Error Ring"() -> ("error out"=w284:errorcluster)
        n115 = call "GetDLLPath.vi"("DllName_32bit"="MHLib" ("name or relative path"), "DllName_64bit"=w273) -> ("file exists?"=w286:bool, "DLLPath"=w287:path)  [unwired: 8 in]
        n116 = global write "MH_DllPath_global.vi" "DllPath"(w287) -> ()
        n117 = Build Array (concatenate)(w309, w308) -> (w260:T8[])
        n118 = Select(t=errorcluster {"status"=FALSE, "code"=0, "source"=""} ("error IO"), s=w286, f=w284) -> (s? t:f=w290:errorcluster)
        n119 = property on="AllChannels" class="Clust (strict)"("Val(Sgnl)"=T2 {"Enable"=TRUE, "Offset"=0, "Level"=20, "Edge"=1, "DeadTime"=1000, "UseDeadTime"=FALSE, "SetEnableAllChan"=TRUE, "SetEdgeAllChan"=TRUE, "SetLevelAllChan"=TRUE, "SetOffsetAllChan"=TRUE, "SetUseDTAllChan"=TRUE, "SetDeadTAllChan"=TRUE} ("AllChannels")) -> ()  [unwired: 2 in, 2 out]
        n120 = global read "MH_LibVersion_global.vi" "Library Version"() -> (w282:string)
        n121 = property on="HistoGraph" class="WFGraph (strict)"("LegPlotMin"=u32 8 ("Legend:Plot Minimum")) -> ()  [unwired: 2 in, 2 out]
        n122 = property on="Scale" class="RadioBtnsControl (strict)"("Val(Sgnl)"=enum32{"Item 0", "Item 1"}."Item 0" ("Value (Signaling)")) -> ()  [unwired: 2 in, 2 out]
        n123 = call "InitMH_UIThread.vi"("error in (no error)"=w290, "Mode"=w274, "refsource"=w283, "Library Version"=w282) -> ("error out"=w310:errorcluster, "Init Info"=w312:T5, "DevIdx"=w311:i32)  [unwired: 5 in]
        n124 = local write "Binning"(w303) -> ()
        n125 = local write "StopOvl."(w299) -> ()
        n126 = local write "Start"(w297) -> ()
        n127 = local write "SyncOffset"(w306) -> ()
        n128 = local write "SyncEdge"(w305) -> ()
        n129 = local write "UseDeadTime"(w272) -> ()
        n130 = local write "HistoOffset"(w302) -> ()
        n131 = local write "HistoLength"(w300) -> ()
        n132 = local write "OvlLevel"(w298) -> ()
        n133 = local write "Run continuously"(enum32{"Running Mode", "Item 1"}."Running Mode" ("Run continuously")) -> ()
        n134 = local write "SyncDivider"(w307) -> ()
        n135 = local write "SyncLevel"(w304) -> ()
        n136 = local write "SyncDeadTime"(w271) -> ()
        n137 = local write "AcqTime"(w301) -> ()
        n138 = Bundle By Name(cluster=w294, "DevIdx"=w311, "Init Info"=w312, "Status"="Initialized!") -> (w293:T4)
        n139 = Unbundle By Name(w293) -> ("Init Info.Bin Steps"=w292:i32, "Init Info.Base Resolution"=w264:dbl, "Init Info.nchannels"=w269:i32)
        n140 = Initialize Array(u32 0, w269, 1024 ("dimension size")) -> (w276:u32[][])
        n141 = call "MH_InitChannels.vi"("nchannels"=w269) -> ("SetInpChan"=w267:T6[], "Channels"=w268:T10[])  [unwired: 9 in]
        n142 = To Unsigned Long Integer(number=w264) -> (unsigned 32bit integer=w265:u32)
        n143 = Divide(x=w264, y=1000.0) -> (x/y=w277:dbl)
        n144 = property on="Offset" class="DigNum (strict)"("Increment"=w264) -> ()  [unwired: 2 in, 2 out]
        n145 = property on="SyncOffset" class="DigNum (strict)"("Increment"=w264) -> ()  [unwired: 2 in, 2 out]
        n146 = property on="Offset" class="DigNum (strict)"("Increment"=w264) -> ()  [unwired: 2 in, 2 out]
        n147 = call "MH_CalcBinningValues.vi"("BaseResolution"=w265, "Bin Steps"=w292) -> ("BinningValues"=w296:cluster{"String":string, "Value":i32}[])  [unwired: 9 in]
        n148 = Bundle(0.0, w277, w276) -> (w270:cluster{dbl, dbl, u32[][]})  [unwired: 1 in]
        n149 = for {
          N: w269 -> [_]
          tunnel: w270 -> [w320]
          i -> [w322]
          n150 = Increment(x=w322) -> (x+1=w321:i32)
          n151 = Format Into String(format string="Ch.%d", w321) -> (resulting string=w323:string)  [unwired: 2 in, 1 out]
          n152 = property on="HistoGraph" class="WFGraph (strict)"("Value"=w320, "Active Plot"=w322, "Plot.Plot Name"=w323) -> ()  [unwired: 2 in, 2 out]
        }
        n153 = property on="Binning" class="Ring (strict)"("StringsAndValues[]"=w296) -> ()  [unwired: 2 in, 2 out]
        n154 = local write "Channels"(w268) -> ()
        n155 = Bundle By Name(cluster=w293, "Channels"=w268, "SetInpChan"=w267, "SyncDivider"=w307, "SyncOffset"=w306, "SyncEdge"=w305, "SyncLevel"=w304, "UseDeadTime"=w272, "SyncDeadTime"=w271, "Binning"=w303, "HistoOffset"=w302, "AcqTime"=w301, "HistoLen"=w300, "StopOvl."=w299, "OvlLevel"=w298, "StartMeas"=w297, "Run cont."=FALSE, "max value"=u32[] [0, 0, 0, 0]) -> (w289:T4)
      }
      frame "SetInpChan" {
        n156 = call "SetInputChannels.vi"("MH_UIThread_Data"=w327) -> ("error out"=w326:errorcluster)  [unwired: 10 in]
      }
      frame "SetSyncDivider" {
        n157 = call "SetSyncDivider.vi"("MH_UIThread_Data"=w330) -> ("error out"=w329:errorcluster)  [unwired: 10 in]
      }
      frame "SetSyncTrg" {
        n158 = Unbundle By Name(w336) -> ("DevIdx"=w334:i32, "SyncLevel"=w332:i32, "SyncEdge"=w333:i32)
        n159 = call "MH_SetSyncEdgeTrg.vi"("edge"=w333, "level"=w332, "devidx"=w334) -> ("error out"=w335:errorcluster)  [unwired: 7 in, 1 out]
      }
      frame "SetSyncDeadTime" {
        w340 = 32  # FEATURE_PROG_TD
        n160 = Unbundle By Name(w348) -> ("DevIdx"=w346:i32, "UseDeadTime"=w344:bool, "SyncDeadTime"=w345:i32, "Init Info.features"=w339:i32)
        n161 = Boolean To (0,1)(Boolean=w344) -> (0, 1=w343:i16)
        n162 = And(x=w339, y=w340) -> (x .and. y?=w341:i32)
        n163 = To Long Integer(number=w343) -> (32bit integer=w342:i32)
        n164 = Not Equal To 0?(x=w341) -> (x != 0?=w338:bool)
        n165 = case shown="False" w338 {
          tunnel: [_ w352] -> w347
          tunnel: w346 -> [_ w351]
          tunnel: w345 -> [_ w350]
          tunnel: w342 -> [_ w349]
          frame False {
          }
          frame True {
            n166 = call "MH_SetSyncDeadTime.vi"("deadtime"=w350, "on"=w349, "devidx"=w351) -> ("error out"=w352:errorcluster)  [unwired: 7 in, 1 out]
          }
        }
      }
      frame "SetSyncOffset" {
        n167 = Unbundle By Name(w357) -> ("DevIdx"=w355:i32, "SyncOffset"=w354:i32)
        n168 = call "MH_SetSyncChannelOffset.vi"("Offset"=w354, "devidx"=w355) -> ("error out"=w356:errorcluster)  [unwired: 8 in, 1 out]
      }
      frame "SetBinning" {
        # "When binning is changed the new resolution is querried"
        n169 = Unbundle By Name(w364) -> ("DevIdx"=w362:i32, "Binning"=w361:i32)
        n170 = call "MH_SetBinning.vi"("Binning"=w361, "devidx"=w362) -> ("error out"=w363:errorcluster)  [unwired: 8 in, 1 out]
        n171 = Build Array (concatenate)(MH_UIThread_Cmds_T2."GetResolution", w360) -> (w358:T8[])
      }
      frame "SetHistoOffset" {
        n172 = Unbundle By Name(w369) -> ("DevIdx"=w367:i32, "HistoOffset"=w366:i32)
        n173 = call "MH_SetOffset.vi"("Offset"=w366, "devidx"=w367) -> ("error out"=w368:errorcluster)  [unwired: 8 in, 1 out]
      }
      frame "SetHistoLen" {
        n174 = Unbundle By Name(w373) -> ("DevIdx"=w375:i32, "HistoLen"=w374:i32)
        n175 = call "MH_SetHistoLen.vi"("lencode"=w374, "devidx"=w375) -> ("error out"=w376:errorcluster, "actuallen"=w371:i32)  [unwired: 7 in, 1 out]
        n176 = Bundle By Name(cluster=w373, "HistoLength"=w371) -> (w372:T4)
      }
      frame "SetStopOvl" {
        n177 = Unbundle By Name(w382) -> ("DevIdx"=w380:i32, "StopOvl."=w379:bool, "OvlLevel"=w378:u32)
        n178 = call "MH_SetStopOverflow.vi"("stopcount"=w378, "StopOnOverflow"=w379, "devidx"=w380) -> ("error out"=w381:errorcluster)  [unwired: 7 in, 1 out]
      }
      frame "GetAllRates" {
        # "An alternative to GetRates"
        n179 = Unbundle By Name(w393) -> ("DevIdx"=w390:i32, "Init Info.nchannels"=w387:i32)
        n180 = call "MH_AllocateCntRateBuffer.vi"("NumChan"=w387) -> ("Buffer"=w388:i32[])  [unwired: 10 in]
        n181 = call "MH_GetAllCountRates.vi"("cntrates_buf"=w388, "devidx"=w390) -> ("error out"=w389:errorcluster, "cntrates"=w385:i32[], "syncrate"=w386:i32)  [unwired: 6 in, 1 out]
        n182 = Build Array (concatenate)(w386, w385) -> (→"CountRates":i32[])
        n183 = Format Into String(format string="Sync Rate: %d cps\n", w386) -> (resulting string=→"SyncRate":string)  [unwired: 2 in, 1 out]
      }
      frame "GetRates" {
        # "An alternative to GetAllRates"
        n184 = Unbundle By Name(w404) -> ("Init Info.nchannels"=w399:i32, "Channels"=w401:T3[], "DevIdx"=w400:i32)
        n185 = call "MH_GetSyncRate.vi"("devidx"=w400) -> ("error out"=w397:errorcluster, "syncrate"=w396:i32)  [unwired: 8 in, 1 out]
        n186 = Format Into String(format string="Sync Rate: %d cps\n", w396) -> (resulting string=w398:string)  [unwired: 2 in, 1 out]
        n187 = for {
          N: w399 -> [_]
          tunnel: w400 -> [w410]
          tunnel: [w407] -> w395 mode=indexing
          shift-right: [w409] -> w403
          shift-left: w397 -> [w411]
          tunnel: w401 -> [w406] mode=indexing
          i -> [w408]
          n188 = Unbundle By Name(w406) -> ("Enable"=w405:bool)
          n189 = case shown="True" w405 {
            tunnel: w411 -> [w412 w417]
            tunnel: w410 -> [_ w416]
            tunnel: [w412 w415] -> w409
            tunnel: w408 -> [_ w414]
            tunnel: [_ w413] -> w407
            frame False {
            }
            frame True {
              n190 = call "MH_GetCountRate.vi"("error in (no error)"=w417, "Channel"=w414, "devidx"=w416) -> ("error out"=w415:errorcluster, "rate"=w413:i32)  [unwired: 6 in, 1 out]
            }
          }
        }
        n191 = local write "CountRates"(w395) -> ()
        n192 = local write "SyncRate"(w398) -> ()
      }
      frame "StartMeas" {
        n193 = Unbundle By Name(w421) -> ("AcqTime"=w424:i32, "DevIdx"=w425:i32)
        n194 = call "MH_ClearHistMem.vi"("devidx"=w425) -> ("error out"=w426:errorcluster)  [unwired: 9 in, 1 out]
        n195 = call "MH_StartMeas.vi"("error in (no error)"=w426, "tacq"=w424, "devidx"=w425) -> ("error out"=w427:errorcluster)  [unwired: 7 in, 1 out]
        n196 = Build Array (concatenate)(w423, MH_UIThread_Cmds_T2."GetAllHistos") -> (w418:T8[])
        n197 = Bundle By Name(cluster=w421, "max value"=u32[] [0, 0, 0, 0]) -> (w420:T4)
      }
      frame "StopMeas" {
        n198 = Unbundle By Name(w433) -> ("Run cont."=w429:bool, "DevIdx"=w434:i32)
        n199 = call "MH_StopMeas.vi"("devidx"=w434) -> ("error out"=w435:errorcluster)  [unwired: 9 in, 1 out]
        n200 = case shown="False" w429 {
          tunnel: w433 -> [w439 w441]
          tunnel: [w438 w441] -> w432
          tunnel: [w436 w440] -> w431
          frame False {
            w436 = T8[] [enum."GetAllHistos"] items=["Idle", "Init", "SetInpChan", "SetSyncDivider", "SetSyncTrg", "SetSyncOffset", "SetSyncDeadTime", "SetBinning", "SetHistoOffset", "SetHistoLen", "SetStopOvl", "SetBitShift", "SetHistoAcqTime", "GetRates", "GetAllRates", "StartMeas", "StopMeas", "AbortMeas", "GetResolution", "GetHistos", "GetAllHistos", "ReadFiFo", "WriteStatus", "Resize", "EnableControls", "DisableControls", "Error", "Exit", "Acquire", "InitAcquisition"]
            w437 = FALSE ("StartMeas")
            n201 = Bundle By Name(cluster=w439, "StartMeas"=w437) -> (w438:T4)
            n202 = local write "Start"(w437) -> ()
          }
          frame True {
            w440 = T8[] [enum."GetAllHistos", enum."StartMeas"] items=["Idle", "Init", "SetInpChan", "SetSyncDivider", "SetSyncTrg", "SetSyncOffset", "SetSyncDeadTime", "SetBinning", "SetHistoOffset", "SetHistoLen", "SetStopOvl", "SetBitShift", "SetHistoAcqTime", "GetRates", "GetAllRates", "StartMeas", "StopMeas", "AbortMeas", "GetResolution", "GetHistos", "GetAllHistos", "ReadFiFo", "WriteStatus", "Resize", "EnableControls", "DisableControls", "Error", "Exit", "Acquire", "InitAcquisition"]
          }
        }
        n203 = Build Array (concatenate)(w430, w431) -> (w428:T8[])
      }
      frame "AbortMeas" {
        w445 = T8[] [enum."GetAllHistos"] items=["Idle", "Init", "SetInpChan", "SetSyncDivider", "SetSyncTrg", "SetSyncOffset", "SetSyncDeadTime", "SetBinning", "SetHistoOffset", "SetHistoLen", "SetStopOvl", "SetBitShift", "SetHistoAcqTime", "GetRates", "GetAllRates", "StartMeas", "StopMeas", "AbortMeas", "GetResolution", "GetHistos", "GetAllHistos", "ReadFiFo", "WriteStatus", "Resize", "EnableControls", "DisableControls", "Error", "Exit", "Acquire", "InitAcquisition"]
        w443 = FALSE ("StartMeas")
        n204 = Unbundle By Name(w447) -> ("DevIdx"=w448:i32)
        n205 = call "MH_StopMeas.vi"("devidx"=w448) -> ("error out"=w449:errorcluster)  [unwired: 9 in, 1 out]
        n206 = Bundle By Name(cluster=w447, "StartMeas"=w443) -> (w446:T4)
        n207 = local write "Start"(w443) -> ()
        n208 = Build Array (concatenate)(w444, w445) -> (w442:T8[])
      }
      frame "GetResolution" {
        # "Resolution in ns"
        # "Gets resolution in ps"
        # "Resolution is saved in UIThread Data cluster in ns"
        n209 = Unbundle By Name(w455) -> ("DevIdx"=w457:i32)
        n210 = call "MH_GetResolution.vi"("devidx"=w457) -> ("error out"=w456:errorcluster, "resolution"=w453:dbl)  [unwired: 8 in, 1 out]
        n211 = Divide(x=w453, y=1000.0) -> (x/y=w451:dbl)
        n212 = Bundle By Name(cluster=w455, "Resolution"=w451) -> (w454:T4)
      }
      frame "GetAllHistos" {
        w488 = 1  # FLAG_OVERFLOW
        # "Provides a buffer (U32-array of length 'HistoLength' x nchannels) for all histograms."
        # "An alternative to GetHistos"
        n213 = Unbundle By Name(w475) -> ("Resolution"=w471:dbl, "DevIdx"=w479:i32, "HistoLength"=w482:i32, "Init Info.nchannels"=w483:i32, "max value"=w467:u32[], "CoincidenceArray"=w462:dbl[][])
        n214 = call "MH_AllocateAllHistoBuffer.vi"("NumChan"=w483, "HistoLength"=w482) -> ("Buffer"=w480:u32[])  [unwired: 9 in]
        n215 = call "MH_GetAllHistograms.vi"("Chcount"=w480, "devidx"=w479) -> ("error out"=w477:errorcluster, "Histograms"=w478:u32[])  [unwired: 7 in, 1 out]
        n216 = Reshape Array(w478, w483, w482) -> (w481:u32[][])
        n217 = call "MH_GetFlags.vi"("error in (no error)"=w477) -> ("error out"=w473:errorcluster, "flags"=w487:i32)  [unwired: 8 in, 1 out]
        n218 = And(x=w488, y=w487) -> (x .and. y?=w489:i32)
        n219 = Not Equal To 0?(x=w489) -> (x != 0?=→"OverFlow":bool)
        n220 = for {
          N: 4 -> [_]
          tunnel: [w508] -> w466 mode=indexing
          shift-right: [w510] -> w484
          shift-left: "Total Counts:\t\t" -> [w509]
          tunnel: w481 -> [w508] mode=indexing
          i -> [w514]
          n221 = Add Array Elements(numeric array=w508) -> (sum=w511:u32)
          n222 = Increment(x=w514) -> (x+1=w512:i32)
          n223 = Format Into String(format string="Ch.%2d: %d cnts.\t\t", initial string=w509, w512, w511) -> (resulting string=w510:string)  [unwired: 1 in, 1 out]
        }
        n224 = call "CalcRate.vi"("Refresh(ms)"="Refresh(ms)") -> ("Rate / Hz"=w465:dbl)  [unwired: 8 in, 2 out]
        n225 = Format Into String(format string="Readout Rate: %.1f Hz\\t\\t", w465) -> (resulting string=w493:string)  [unwired: 2 in, 1 out]
        n226 = for {
          tunnel: w471 -> [w503]
          tunnel: [w495] -> w463 mode=indexing
          tunnel: w467 -> [w502] mode=indexing
          tunnel: w466 -> [w499] mode=indexing
          tunnel: w465 -> [w498]
          tunnel: [w497] -> w464 mode=indexing
          n227 = Array Max & Min(array=w499) -> (max value=w497:u32, max index (indices)=w500:i32)  [unwired: 2 out]
          n228 = Subtract(x=w497, y=w502) -> (x-y=w501:u32)
          n229 = Multiply(x=w500, y=w503) -> (x*y=→"x*y":dbl)
          n230 = disable-structure shown="Enabled" {
            disable-tunnel: w501 -> [w506 w507]
            disable-tunnel: w498 -> [w505 _]
            disable-tunnel: [w504 w507] -> w495
            frame Disabled {
              n231 = Multiply(x=w506, y=w505) -> (x*y=w504:dbl)
            }
            frame Enabled {
            }
          }
        }
        n232 = Concatenate Strings(w493, w484) -> (w492:string)
        n233 = Bundle(0.0, "Resolution"=w471, "Histograms"=w466) -> (→"HistoGraph":T1)  [unwired: 1 in]
        n234 = local write "Status"(w492) -> ()
        n235 = Build Array (concatenate)(w462, w463) -> (w459:dbl[][])
        n236 = Send Notification(notification=w459, notifier=w469) -> (error out=w468:errorcluster)  [unwired: 1 in, 1 out]
        n237 = call "GetLastnElemsfromArray.vi"("array"=w459, "y"="Monitor Range") -> ("deleted portion"=w460:dbl[][])
        n238 = Merge Errors(w473, w468) -> (w472:errorcluster)
        n239 = Bundle By Name(cluster=w475, "max value"=w464, "CoincidenceArray"=w460) -> (w474:T4)
      }
      frame "GetHistos" {
        w525 = 1  # FLAG_OVERFLOW
        # "Provides a buffer (U32-array of length 'HistoLength') for histograms."
        # "An alternative to GetAllHistos"
        n240 = Unbundle By Name(w539) -> ("Resolution"=w536:dbl, "Init Info.nchannels"=w518:i32, "Channels"=w519:T3[], "DevIdx"=w538:i32, "HistoLength"=w537:i32)
        n241 = call "MH_AllocateHistoBuffer.vi"("HistoLength"=w537) -> ("Buffer"=w530:u32[])  [unwired: 10 in]
        n242 = for {
          N: w518 -> [_]
          tunnel: w538 -> [w552]
          tunnel: [w540] -> w528 mode=indexing
          tunnel: w530 -> [w550]
          shift-right: [w551] -> w527
          shift-left: errorcluster {"status"=FALSE, "code"=0, "source"=""} ("error IO") -> [w544]
          shift-right: [w545] -> w521
          shift-left: "Total Counts:\t\t" -> [w543]
          tunnel: w519 -> [w542] mode=indexing
          i -> [w549]
          n243 = Unbundle By Name(w542) -> ("Enable"=w541:bool)
          n244 = case shown="True" w541 {
            tunnel: w552 -> [_ w560]
            tunnel: [w553 w559] -> w551
            tunnel: w550 -> [w554 w558]
            tunnel: [w554 w557] -> w540
            tunnel: w549 -> [_ w556]
            tunnel: w544 -> [w553 w555]
            frame False {
            }
            frame True {
              n245 = call "MH_GetHistogram.vi"("Chcount"=w558, "error in (no error)"=w555, "channel"=w556, "devidx"=w560) -> ("error out"=w559:errorcluster, "Histogram"=w557:u32[])  [unwired: 5 in, 1 out]
            }
          }
          n246 = Add Array Elements(numeric array=w540) -> (sum=w546:u32)
          n247 = Increment(x=w549) -> (x+1=w547:i32)
          n248 = Format Into String(format string="Ch.%2d: %d cnts.\t\t", initial string=w543, w547, w546) -> (resulting string=w545:string)  [unwired: 1 in, 1 out]
        }
        n249 = call "CalcRate.vi"("Refresh(ms)"=u32 500) -> ("Rate / Hz"=w534:dbl)  [unwired: 8 in, 2 out]
        n250 = Format Into String(format string="Readout Rate: %.1f Hz\\t\\t", w534) -> (resulting string=w532:string)  [unwired: 2 in, 1 out]
        n251 = Concatenate Strings(w532, w521) -> (w531:string)
        n252 = Bundle(0.0, "Resolution"=w536, "Histogram"=w528) -> (w516:T14)  [unwired: 1 in]
        n253 = local write "HistoGraph"(w516) -> ()
        n254 = local write "Status"(w531) -> ()
        n255 = call "MH_GetFlags.vi"("error in (no error)"=w527) -> ("error out"=w535:errorcluster, "flags"=w524:i32)  [unwired: 8 in, 1 out]
        n256 = And(x=w525, y=w524) -> (x .and. y?=w526:i32)
        n257 = Not Equal To 0?(x=w526) -> (x != 0?=w517:bool)
        n258 = local write "OverFlow"(w517) -> ()
      }
      frame "WriteStatus" {
        n259 = Unbundle By Name(w563) -> ("Status"=→"Status":string)
      }
      frame "EnableControls" {
        n260 = property class="VI"() -> ("Panel"=w568:refnum<vi>)  [unwired: 2 in, 2 out]
        n261 = property class="Pnl"(reference=w568) -> ("Decos[]"=w569:refnum<vi>[])  [unwired: 1 in, 2 out]
        n262 = property class="Pnl"(reference=w568) -> ("Controls[]"=w567:refnum<vi>[])  [unwired: 1 in, 2 out]
        n263 = for {
          tunnel: w569 -> [w572] mode=indexing
          tunnel: TRUE -> [w571]
          n264 = property class="Decor"(reference=w572, "Visible"=w571) -> ()  [unwired: 1 in, 2 out]
        }
        n265 = for {
          tunnel: w567 -> [w575] mode=indexing
          tunnel: T9."Enabled" ("Disabled") -> [w574]
          tunnel: [w573] -> _
          n266 = property class="Ctl"(reference=w575, "DisabledEnum"=w574) -> (error out=w573:errorcluster)  [unwired: 1 in, 1 out]
        }
      }
      frame "DisableControls" {
        n267 = property class="VI"() -> ("Panel"=w580:refnum<vi>)  [unwired: 2 in, 2 out]
        n268 = property class="Pnl"(reference=w580) -> ("Decos[]"=w581:refnum<vi>[])  [unwired: 1 in, 2 out]
        n269 = property class="Pnl"(reference=w580) -> ("Controls[]"=w579:refnum<vi>[])  [unwired: 1 in, 2 out]
        n270 = for {
          tunnel: w581 -> [w584] mode=indexing
          tunnel: FALSE -> [w583]
          n271 = property class="Decor"(reference=w584, "Visible"=w583) -> ()  [unwired: 1 in, 2 out]
        }
        n272 = for {
          tunnel: w579 -> [w587] mode=indexing
          tunnel: T9."Disabled and Grayed Out" ("Disabled") -> [w586]
          tunnel: [w585] -> _
          n273 = property class="Ctl"(reference=w587, "DisabledEnum"=w586) -> (error out=w585:errorcluster)  [unwired: 1 in, 1 out]
        }
      }
      frame "Error" {
        w588 = T8[] [enum."Exit"] items=["Idle", "Init", "SetInpChan", "SetSyncDivider", "SetSyncTrg", "SetSyncOffset", "SetSyncDeadTime", "SetBinning", "SetHistoOffset", "SetHistoLen", "SetStopOvl", "SetBitShift", "SetHistoAcqTime", "GetRates", "GetAllRates", "StartMeas", "StopMeas", "AbortMeas", "GetResolution", "GetHistos", "GetAllHistos", "ReadFiFo", "WriteStatus", "Resize", "EnableControls", "DisableControls", "Error", "Exit", "Acquire", "InitAcquisition"]
        w591 = T15 1 items=["no dialog", "OK message", "continue or stop message", "OK message + warnings", "continue/stop + warnings"] ("type of dialog (OK msg:1)")
        # "Error case: If an error occures the user is informed and the programm terminates. Add your own code to handle error events (e.g. exception lists, etc.)"
        n274 = call <vilib>:"Simple Error Handler.vi"("type of dialog (OK msg:1)"=w591, "error in (no error)"=w590) -> ()  [unwired: 3 in, 5 out]
      }
      frame "Exit" {
        n275 = Unbundle By Name(w599) -> ("DevIdx"=w598:i32)
        n276 = call "MH_CloseDevice.vi"("devidx"=w598) -> ("error out"=w595:errorcluster)  [unwired: 9 in, 1 out]
        n277 = Release Notifier(notifier=w593, error in (no error)=w597) -> (error out=w596:errorcluster)  [unwired: 3 out]
        n278 = Merge Errors(w596, w595) -> (w594:errorcluster)
      }
      frame "Acquire" {
        w607 = T12 2 items=["HIST"=0, "T2"=2, "T3"=3] ("Mode")
        w610 = T8[] [enum."DisableControls", enum."Init"] items=["Idle", "Init", "SetInpChan", "SetSyncDivider", "SetSyncTrg", "SetSyncOffset", "SetSyncDeadTime", "SetBinning", "SetHistoOffset", "SetHistoLen", "SetStopOvl", "SetBitShift", "SetHistoAcqTime", "GetRates", "GetAllRates", "StartMeas", "StopMeas", "AbortMeas", "GetResolution", "GetHistos", "GetAllHistos", "ReadFiFo", "WriteStatus", "Resize", "EnableControls", "DisableControls", "Error", "Exit", "Acquire", "InitAcquisition"]
        n279 = Path To String(path="Path") -> (string=w604:string)
        n280 = call "python_acquisition_multiple_in_python.vi"("MH_UIThread_Data"=w602, "FileName"="FileName 2", "mode"=w607, "Number \nof Acquisitions"="Number of Acquisitions", "Directory"=w604) -> ("error out"=w603:errorcluster)  [unwired: 2 in]
        n281 = Build Array (concatenate)(w609, w610) -> (w601:T8[])
      }
      frame "InitAcquisition" {
        n282 = Unbundle By Name(w612) -> ("DevIdx"=w614:i32)
        n283 = call "MH_CloseDevice.vi"("devidx"=w614) -> ("error out"=w613:errorcluster)  [unwired: 9 in, 1 out]
        n284 = Build Array (concatenate)(w615, MH_UIThread_Cmds_T2."Acquire") -> (w611:T8[])
      }
    }
    n285 = call "MH_EnQErrorT2.vi"("error in (no error)"=w11, "Cmds_in"=w7) -> ("error out"=w10:errorcluster, "Array"=w9:T8[])  [unwired: 8 in]
  }
  n286 = while {
    tunnel: w2 -> [w619]
    stop <- w618 stop-if-true
    n287 = Wait on Notification(notifier=w619) -> (notification=→"Waveform Chart":dbl[][], error out=w618:errorcluster)  [unwired: 3 in, 2 out]
  }
